vi "SwissSPAD Live_Save Dataset Sum Preview Images.vi"(6 "Save Preview":bool, 8 "error in (no error)":errorcluster, 9 "G2 Sum":i32[][](array[numeric]), 10 "INT Sum":i32[][](array[numeric]), 11 "HDF5 File Path":path) -> (0 "error out":errorcluster)   [LabVIEW 2021]
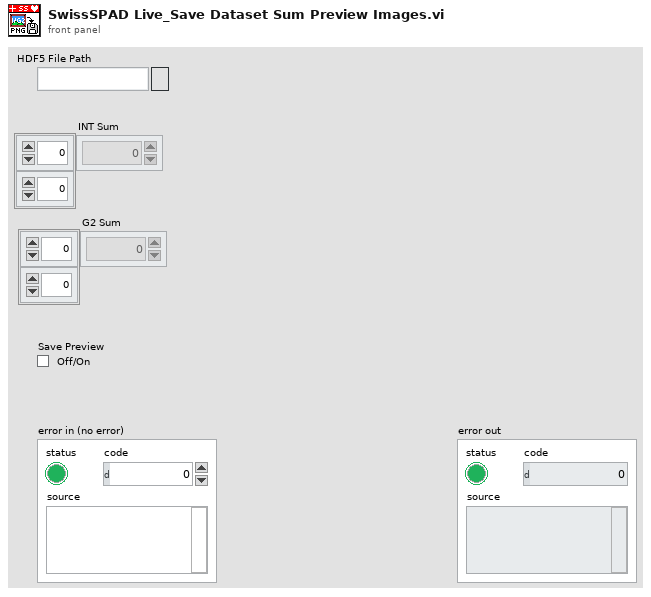
[diagram p1: front panel]
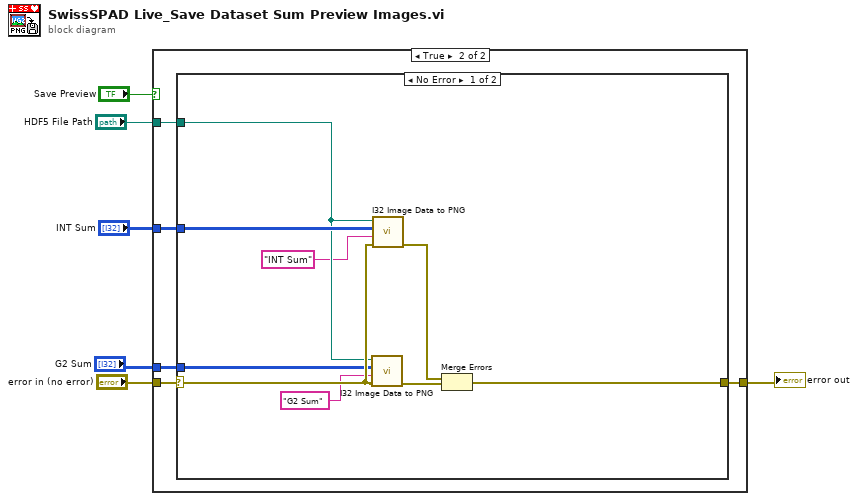
[diagram p0: block diagram]
diagram:
  n1 = case shown="True" "Save Preview" {
    tunnel: "error in (no error)" -> [w7 w12]
    tunnel: [w7 w11] -> w4
    tunnel: "HDF5 File Path" -> [_ w10]
    tunnel: "INT Sum" -> [_ w9]
    tunnel: "G2 Sum" -> [_ w8]
    frame False {
    }
    frame True {
      n2 = case shown="No Error" w12 {
        selector: w12 -> [w19 w22]
        tunnel: [w18 w22] -> w11
        tunnel: w10 -> [w15 _]
        tunnel: w9 -> [w21 _]
        tunnel: w8 -> [w14 _]
        frame No Error {
          n3 = call "I32 Image Data to PNG.vi"("error in (no error)"=w19, "Image Name Suffix"="G2 Sum" ("string"), "Image Data"=w14, "Reference File Path"=w15) -> ("error out"=w17:errorcluster)  [unwired: 5 in, 2 out]
          n4 = call "I32 Image Data to PNG.vi"("error in (no error)"=w19, "Image Name Suffix"="INT Sum" ("string"), "Image Data"=w21, "Reference File Path"=w15) -> ("error out"=w20:errorcluster)  [unwired: 5 in, 2 out]
          n5 = Merge Errors(w20, w17) -> (w18:errorcluster)
        }
        frame Error {
        }
      }
    }
  }
  "error out" <- w4
